vi "test Get Array Element AccessType.vi"(11 "Test Case In":refnum<class "test Electronic Datasheet.lvclass">) -> (0 "error out":errorcluster, 3 "Test Case Out":refnum<class "test Electronic Datasheet.lvclass">)   [LabVIEW 2024, in "test Electronic Datasheet.lvclass"]
uses:
  test Electronic Datasheet.lvclass
  C:/Program Files/National Instruments/LabVIEW 2025/vi.lib/Astemes/LUnit/Test Case.lvclass
  Core/Object Type.ctl
  Core/Access Type.ctl
  <vilib>/Astemes/LUnit/Test Case.lvclass/Test Case.ctl
  <vilib>/Astemes/LUnit/Append Fail Result.vi
  <vilib>/Astemes/LUnit/Append Pass Result.vi
  <vilib>/Astemes/LUnit/Run In UI.vi
  <vilib>/Utility/error.llb/Clear Errors.vi
  Core/OD Sub-Entry/OD Sub-Entry.lvclass
  D:/git/EDS-File-Viewer/Core/OD Entry/OD Entry.lvclass
  Electronic Datasheet/utils/Electronic Datasheet_GetAttributes.vi
  Electronic Datasheet/Electronic Datasheet.lvclass
  <vilib>/Astemes/LUnit/Test Case.lvclass
  Core/Electronic Datasheet.lvlib
  Core/OD Entry/OD Entry.lvclass
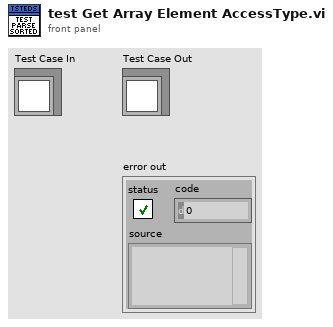
[diagram p1: front panel]
types:
  T1 = typedef "Electronic Datasheet.lvlib/Access Type.ctl" = enum16{"ro", "wo", "rw", "rwr", "rww", "const"}
  T2 = typedef "Electronic Datasheet.lvlib/Object Type.ctl" = u8
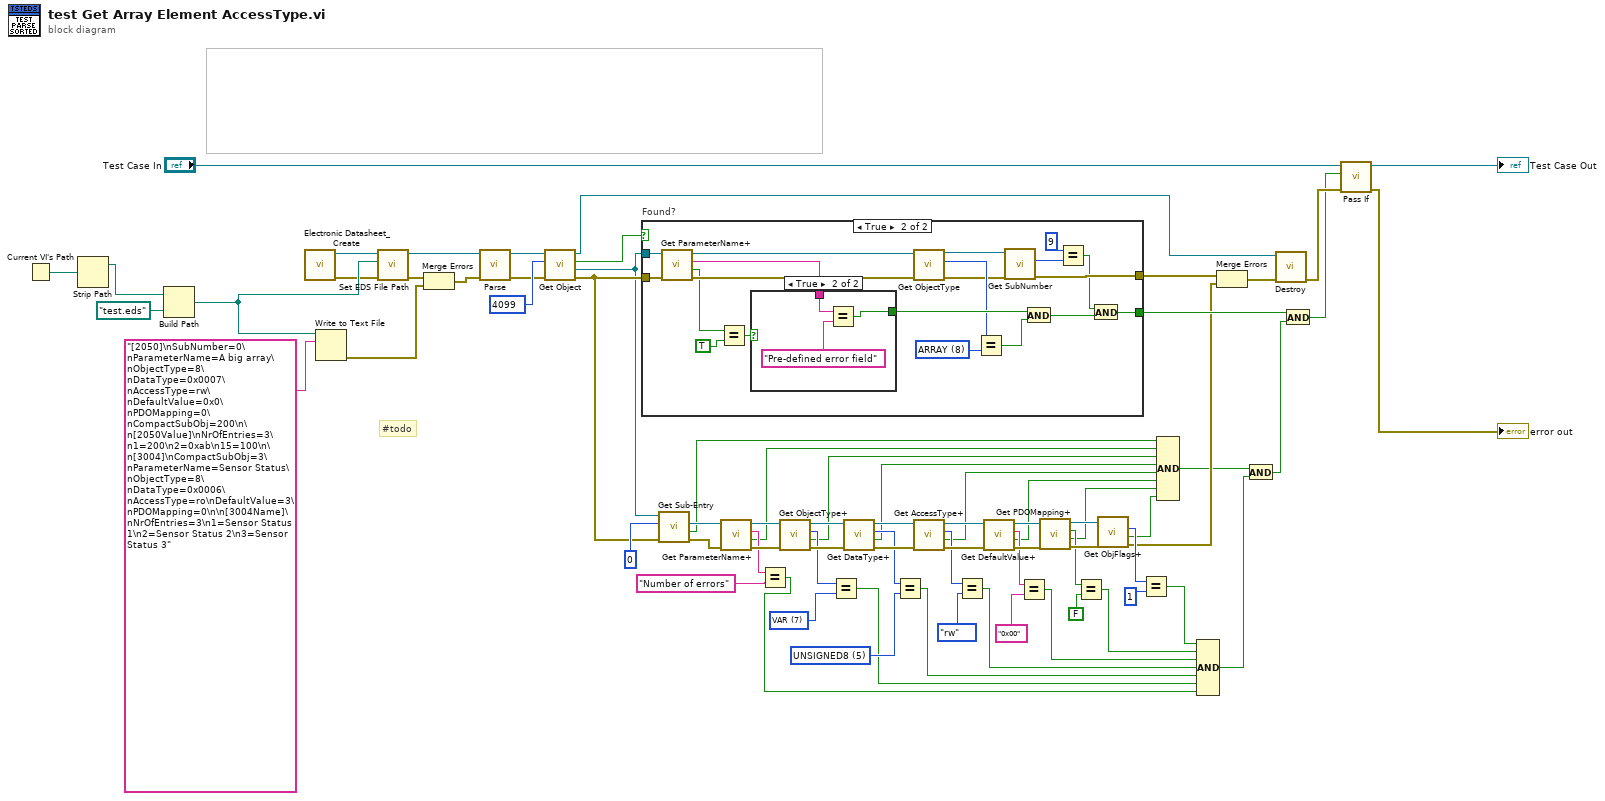
[diagram p0: block diagram]
diagram:
  w43 = u16 5 items=["BOOLEAN"=1, "INTEGER8"=2, "INTEGER16"=3, "INTEGER32"=4, "UNSIGNED8"=5, "UNSIGNED16"=6, "UNSIGNED32"=7, "REAL32"=8, "VISIBLE_STRING"=9, "OCTET_STRING"=10, "UNICODE_STRING"=11, "TIME_OF_DAY"=12, "TIME_DIFFERENCE"=13, "RESERVED1"=14, "DOMAIN"=15, "INTEGER24"=16, "REAL64"=17, "INTEGER40"=18, "INTEGER48"=19, "INTEGER56"=20, "INTEGER64"=21, "UNSIGNED24"=22, "RESERVED2"=23, "UNSIGNED40"=24, "UNSIGNED48"=25, "UNSIGNED56"=26, "UNSIGNED64"=27, "RESERVED3"=28, "RESERVED4"=29, "RESERVED5"=30, "RESERVED6"=31, "PDO_COMMUNICATION_PARAMETER"=32, "PDO_MAPPING"=33, "SDO_PARAMETER"=34, "IDENTITY"=35, "RESERVED7"=36] ("DataType")
  w45 = T2 7 items=["NULL"=0, "DOMAIN"=2, "DEFTYPE"=5, "DEFSTRUCT"=6, "VAR"=7, "ARRAY"=8, "RECORD"=9] ("ObjectType")
  # "#todo"
  n1 = Current VI's Path() -> (path=w70:path)
  n2 = Strip Path(path=w70) -> (stripped path=w66:path)  [unwired: 1 out]
  n3 = Build Path(base path=w66, name or relative path=path "test.eds") -> (appended path=w67:path)
  n4 = call "Electronic Datasheet_Create.vi"() -> ("Error Out"=w9:errorcluster, "reference out"=w10:refnum<class "Electronic Datasheet.lvclass">)  [unwired: 10 in]
  n5 = Write to Text File(file (use dialog)=w67, text="[2050]\nSubNumber=0\nParameterName=A big array\nObjectType=8\nDataType=0x0007\nAccessType=rw\nDefaultValue=0x0\nPDOMapping=0\nCompactSubObj=200\n\n[2050Value]\nNrOfEntries=3\n1=200\n2=0xab\n15=100\n\n[3004]\nCompactSubObj=3\nParameterName=Sensor Status\nObjectType=8\nDataType=0x0006\nAccessType=ro\nDefaultValue=3\nPDOMapping=0\n\n[3004Name]\nNrOfEntries=3\n1=Sensor Status 1\n2=Sensor Status 2\n3=Sensor Status 3") -> (error out=w68:errorcluster)  [unwired: 2 in, 2 out]
  n6 = call "Set EDS File Path.vi"("error in"=w9, "EDS File Path"=w67, "reference in"=w10) -> ("error out"=w1:errorcluster, "reference out"=w71:refnum<class "Electronic Datasheet.lvclass">)  [unwired: 7 in]
  n7 = Merge Errors(w1, w68) -> (w2:errorcluster)
  n8 = call "Parse.vi"("error in"=w2, "reference in"=w71) -> ("error out"=w7:errorcluster, "reference out"=w65:refnum<class "Electronic Datasheet.lvclass">)  [unwired: 8 in]
  n9 = call "Get Object.vi"("error in"=w7, "Index"=u16 4099 ("Numeric"), "reference in"=w65) -> ("error out"=w6:errorcluster, "OD Entry"=w3:refnum<class "OD Entry.lvclass">, "Found?"=w4:bool, "reference out"=w5:refnum<class "Electronic Datasheet.lvclass">)  [unwired: 5 in]
  n10 = case "Found?" shown="True" w4 {
    selector: w4 -> [w75 _]
    tunnel: w3 -> [_ w96]
    tunnel: w6 -> [w76 w95]
    tunnel: [w75 w79] -> w63
    tunnel: [w76 w83] -> w61
    frame False {
    }
    frame True {
      w87 = T2 8 items=["NULL"=0, "DOMAIN"=2, "DEFTYPE"=5, "DEFSTRUCT"=6, "VAR"=7, "ARRAY"=8, "RECORD"=9] ("y")
      n11 = call "Get ParameterName+.vi"("Error In"=w95, "reference in"=w96) -> ("Error Out"=w89:errorcluster, "Defined?"=w77:bool, "ParameterName"=w93:string, "reference out"=w90:refnum<class "OD Entry.lvclass">)  [unwired: 6 in]
      n12 = Equal?(x=w77, y=TRUE) -> (x = y?=w92:bool)
      n13 = case shown="True" w92 {
        selector: w92 -> [w97 _]
        tunnel: w93 -> [_ w100]
        tunnel: [w97 w98] -> w91
        frame False {
        }
        frame True {
          n14 = Equal?(x=w100, y="Pre-defined error field") -> (x = y?=w98:bool)
        }
      }
      n15 = call "Get ObjectType.vi"("Error In"=w89, "reference in"=w90) -> ("Error Out"=w84:errorcluster, "ObjectType"=w88:T2, "reference out"=w82:refnum<class "OD Entry.lvclass">)  [unwired: 7 in]
      n16 = Equal?(x=w88, y=w87) -> (x = y?=w85:bool)
      n17 = call "Get SubNumber.vi"("Error In"=w84, "reference in"=w82) -> ("Error Out"=w83:errorcluster, "SubNumber"=w81:u8)  [unwired: 7 in, 1 out]
      n18 = And(x=w91, y=w85) -> (x .and. y?=w86:bool)
      n19 = Equal?(x=u8 9, y=w81) -> (x = y?=w78:bool)
      n20 = And(x=w78, y=w86) -> (x .and. y?=w79:bool)
    }
  }
  n21 = call "Get Sub-Entry.vi"("Error In"=w6, "Sub-Index"=u8 0, "reference in"=w3) -> ("Error Out"=w59:errorcluster, "Found?"=w47:bool, "OD Sub-Entry"=w60:refnum<class "OD Sub-Entry.lvclass">)  [unwired: 5 in, 1 out]
  n22 = call "Get ParameterName+.vi"("Error In"=w59, "reference in"=w60) -> ("Error Out"=w58:errorcluster, "Defined?"=w17:bool, "ParameterName"=w49:string, "reference out"=w57:refnum<class "OD Sub-Entry.lvclass">)  [unwired: 6 in]
  n23 = Equal?(x=w49, y="Number of errors") -> (x = y?=w24:bool)
  n24 = call "Get ObjectType+.vi"("Error In"=w58, "reference in"=w57) -> ("Error Out"=w55:errorcluster, "Defined?"=w16:bool, "ObjectType"=w46:T2, "reference out"=w56:refnum<class "OD Sub-Entry.lvclass">)  [unwired: 6 in]
  n25 = Equal?(x=w46, y=w45) -> (x = y?=w23:bool)
  n26 = call "Get DataType+.vi"("Error In"=w55, "reference in"=w56) -> ("Error Out"=w52:errorcluster, "Defined?"=w15:bool, "DataType"=w44:u16, "reference out"=w53:refnum<class "OD Sub-Entry.lvclass">)  [unwired: 6 in]
  n27 = Equal?(x=w44, y=w43) -> (x = y?=w22:bool)
  n28 = call "Get AccessType+.vi"("Error In"=w52, "reference in"=w53) -> ("Error Out"=w50:errorcluster, "Defined?"=w14:bool, "AccessType"=w42:T1, "reference out"=w51:refnum<class "OD Sub-Entry.lvclass">)  [unwired: 6 in]
  n29 = Equal?(x=w42, y=Access_Type."rw") -> (x = y?=w21:bool)
  n30 = call "Get DefaultValue+.vi"("Error In"=w50, "reference in"=w51) -> ("Error Out"=w39:errorcluster, "Defined?"=w13:bool, "DefaultValue"=w36:string, "reference out"=w40:refnum<class "OD Sub-Entry.lvclass">)  [unwired: 6 in]
  n31 = Equal?(x=w36, y="0x00") -> (x = y?=w20:bool)
  n32 = call "Get PDOMapping+.vi"("Error In"=w39, "reference in"=w40) -> ("Error Out"=w37:errorcluster, "Defined?"=w12:bool, "PDOMapping"=w34:bool, "reference out"=w38:refnum<class "OD Sub-Entry.lvclass">)  [unwired: 6 in]
  n33 = Equal?(x=w34, y=FALSE) -> (x = y?=w19:bool)
  n34 = call "Get ObjFlags+.vi"("Error In"=w37, "reference in"=w38) -> ("Error Out"=w30:errorcluster, "Defined?"=w11:bool, "ObjFlags"=w32:u32)  [unwired: 6 in, 1 out]
  n35 = Equal?(x=w32, y=u32 1) -> (x = y?=w18:bool)
  n36 = Compound Arithmetic op=AND(w47, w17, w16, w15, w14, w13, w12, w11) -> (w28:bool)
  n37 = Compound Arithmetic op=AND(w18, w19, w20, w21, w22, w23, w24) -> (w25:bool)
  n38 = Merge Errors(w61, w30) -> (w31:errorcluster)
  n39 = And(x=w28, y=w25) -> (x .and. y?=w26:bool)
  n40 = call-dynamic "Destroy.vi"("Error In"=w31, "reference in"=w5) -> ("Error Out"=w62:errorcluster)  [unwired: 8 in, 1 out]
  n41 = And(x=w63, y=w26) -> (x .and. y?=w29:bool)
  n42 = call <vilib>:"Pass If.vi"("error in (no error)"=w62, "Pass?"=w29, "LUnit Test Case In"="Test Case In") -> ("error out"=→"error out":errorcluster, "LUnit Test Case Out"=→"Test Case Out":refnum<class "test Electronic Datasheet.lvclass">)  [unwired: 7 in]
